vi "lj_start.vi"(6 "Period [ms]":i32=500 min=1 max=60000, 8 "error in (no error)":errorcluster, 10 "LabJackRes":T1, 11 "Handle In":i32) -> (0 "error out":errorcluster, 1 "NumReadAddresses":i32, 2 "ScansPerRead Out":i32, 3 "Handle Out":i32)   [LabVIEW 2025, in "LabJackEKG.lvlib"]
uses:
  LabJackEKG.lvlib
  Typedefs/LabJackGlobalResources.ctl
  Typedefs/CounterQueues.ctl
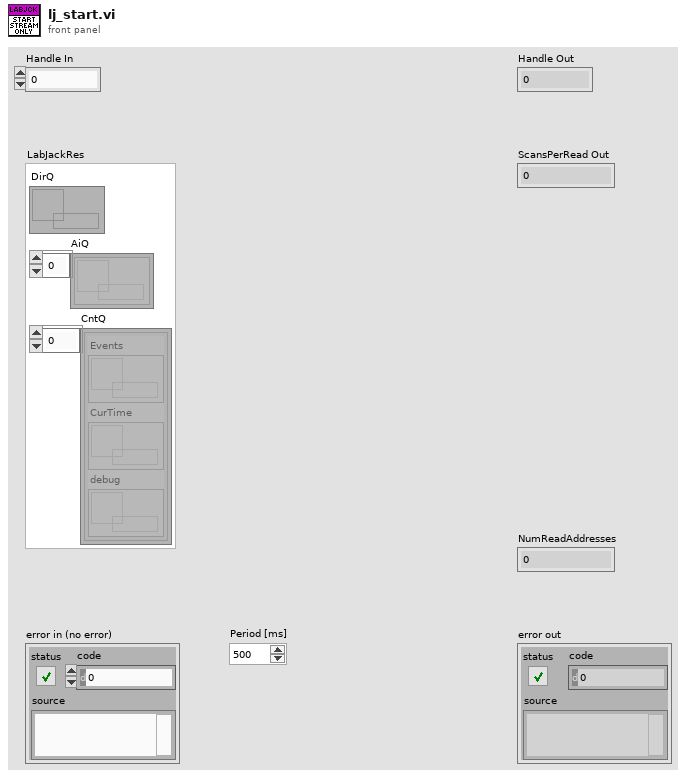
[diagram p1: front panel]
types:
  T1 = typedef "LabJackEKG.lvlib/LabJackGlobalResources.ctl" = cluster{"DirQ":refnum<queue>, "AiQ":refnum<queue>[], "CntQ":T2[]}
  T2 = typedef "LabJackEKG.lvlib/CounterQueues.ctl" = cluster{"Events":refnum<queue>, "CurTime":refnum<queue>, "debug":refnum<queue>}
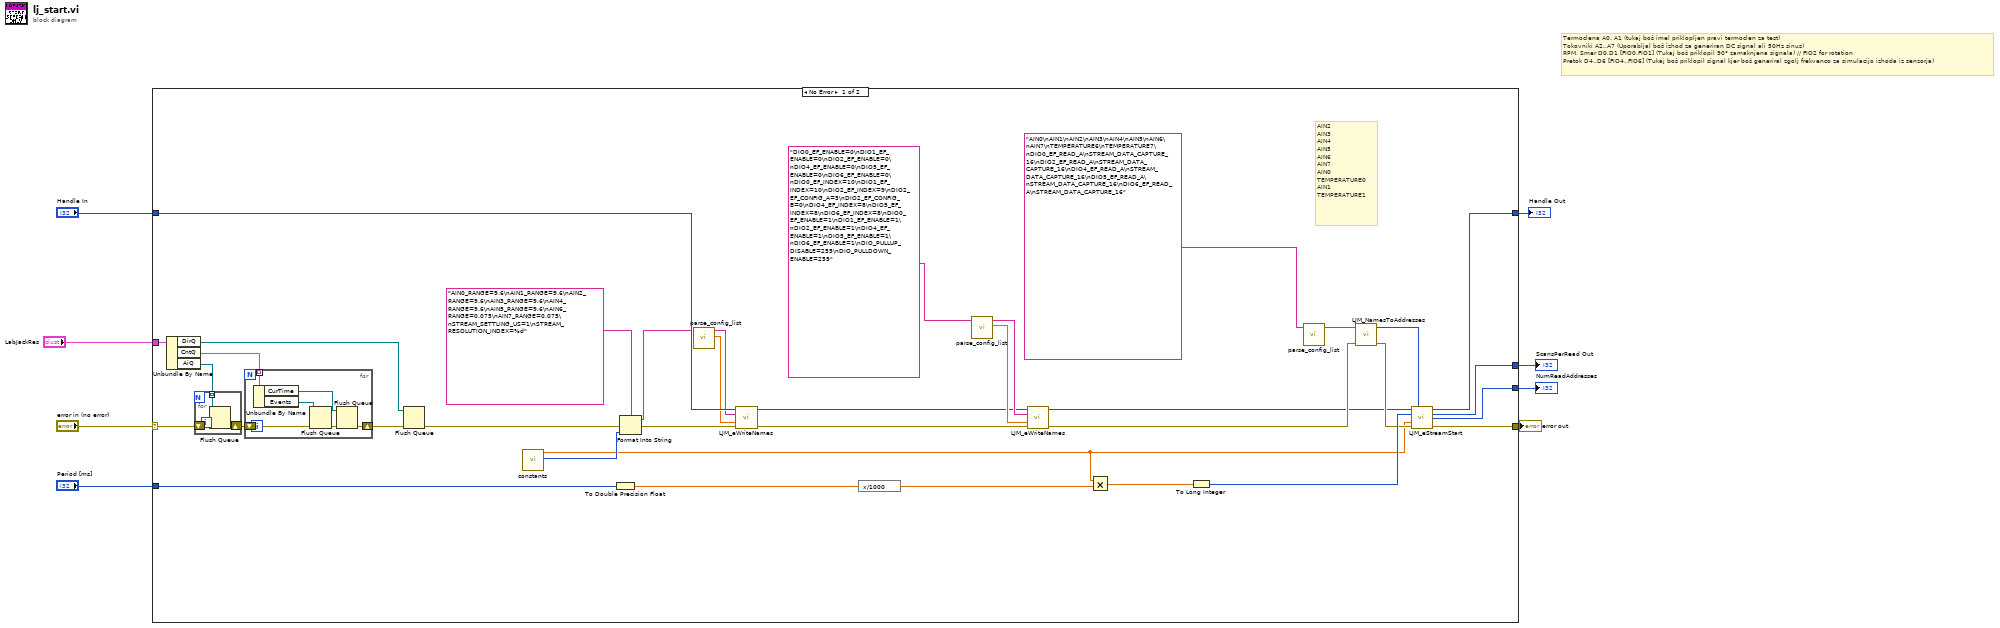
[diagram p0: block diagram]
diagram:
  # "Termoclena A0, A1 (tukaj boš imel priklopljen pravi termoclen za test)\nTokovniki A2..A7 (Uporabljal boš izhod za generiran DC signal ali 50Hz sinus)\nRPM, Smer D0,D1 [FIO0,FIO1] (Tukaj boš priklopil 90° zamaknjena signala) // FIO2 for rotation\nPretok D4..D6 [FIO4..FIO6] (Tukaj boš priklopil signal kjer boš generiral zgolj frekvenco za simulacijo izhoda iz senzorja)"
  n1 = case shown="No Error" "error in (no error)" {
    selector: "error in (no error)" -> [w44 w55]
    tunnel: [w41 w54] -> w8
    tunnel: "Handle In" -> [w43 w54]
    tunnel: [w42 w55] -> w5
    tunnel: [w39 _] -> w4
    tunnel: [w38 _] -> w3
    tunnel: "Period [ms]" -> [w37 _]
    tunnel: "LabJackRes" -> [w23 _]
    frame No Error {
      # "AIN2\nAIN3\nAIN4\nAIN5\nAIN6\nAIN7\nAIN0\nTEMPERATURE0\nAIN1\nTEMPERATURE1"
      n2 = Unbundle By Name(w23) -> ("DirQ"=w19:refnum<queue>, "CntQ"=w18:T2[], "AiQ"=w17:refnum<queue>[])
      n3 = for {
        shift-right: [w52] -> w22
        shift-left: w44 -> [w53]
        tunnel: w17 -> [w51] mode=indexing
        n4 = Flush Queue(queue=w51, error in (no error)=w53) -> (error out=w52:errorcluster)  [unwired: 2 out]
      }
      n5 = for {
        shift-right: [w46] -> w21
        shift-left: w22 -> [w50]
        tunnel: w18 -> [w48] mode=indexing
        n6 = Unbundle By Name(w48) -> ("CurTime"=w45:refnum<queue>, "Events"=w47:refnum<queue>)
        n7 = Flush Queue(queue=w47, error in (no error)=w50) -> (error out=w49:errorcluster)  [unwired: 2 out]
        n8 = Flush Queue(queue=w45, error in (no error)=w49) -> (error out=w46:errorcluster)  [unwired: 2 out]
      }
      n9 = Flush Queue(queue=w19, error in (no error)=w21) -> (error out=w20:errorcluster)  [unwired: 2 out]
      n10 = call "constants.vi"() -> ("Resolution Index"=w13:i32, "Sampling Frequency [Hz]"=w9:dbl)  [unwired: 10 in]
      n11 = To Double Precision Float(number=w37) -> (double precision float=w12:dbl)
      n12 = Format Into String(format string="AIN0_RANGE=9.6\nAIN1_RANGE=9.6\nAIN2_RANGE=9.6\nAIN3_RANGE=9.6\nAIN4_RANGE=9.6\nAIN5_RANGE=9.6\nAIN6_RANGE=0.075\nAIN7_RANGE=0.075\nSTREAM_SETTLING_US=1\nSTREAM_RESOLUTION_INDEX=%d" ("String"), error in=w20, w13) -> (resulting string=w14:string, error out=w16:errorcluster)  [unwired: 1 in]
      n13 = call "parse_config_list.vi"("String"=w14) -> ("Values"=w35:dbl[], "Names"=w36:string[])  [unwired: 9 in]
      n14 = call <vilib>:"LJM_eWriteNames.vi"("Handle In"=w43, "aNames"=w36, "aValuesIn"=w35, "error in"=w16) -> ("Handle Out"=w26:i32, "error out"=w27:errorcluster)  [unwired: 9 in, 1 out]
      n15 = expression code="x/1000"(w12) -> (w11:dbl)
      n16 = call "parse_config_list.vi"("String"="DIO0_EF_ENABLE=0\nDIO1_EF_ENABLE=0\nDIO2_EF_ENABLE=0\nDIO4_EF_ENABLE=0\nDIO5_EF_ENABLE=0\nDIO6_EF_ENABLE=0\nDIO0_EF_INDEX=10\nDIO1_EF_INDEX=10\nDIO2_EF_INDEX=9\nDIO2_EF_CONFIG_A=5\nDIO2_EF_CONFIG_B=0\nDIO4_EF_INDEX=8\nDIO5_EF_INDEX=8\nDIO6_EF_INDEX=8\nDIO0_EF_ENABLE=1\nDIO1_EF_ENABLE=1\nDIO2_EF_ENABLE=1\nDIO4_EF_ENABLE=1\nDIO5_EF_ENABLE=1\nDIO6_EF_ENABLE=1\nDIO_PULLUP_DISABLE=255\nDIO_PULLDOWN_ENABLE=255") -> ("Values"=w30:dbl[], "Names"=w29:string[])  [unwired: 9 in]
      n17 = call <vilib>:"LJM_eWriteNames.vi"("Handle In"=w26, "aNames"=w29, "aValuesIn"=w30, "error in"=w27) -> ("Handle Out"=w25:i32, "error out"=w28:errorcluster)  [unwired: 9 in, 1 out]
      n18 = Multiply(x=w9, y=w11) -> (x*y=w10:dbl)
      n19 = To Long Integer(number=w10) -> (32bit integer=w40:i32)
      n20 = call "parse_config_list.vi"("String"="AIN0\nAIN1\nAIN2\nAIN3\nAIN4\nAIN5\nAIN6\nAIN7\nTEMPERATURE6\nTEMPERATURE7\nDIO0_EF_READ_A\nSTREAM_DATA_CAPTURE_16\nDIO2_EF_READ_A\nSTREAM_DATA_CAPTURE_16\nDIO4_EF_READ_A\nSTREAM_DATA_CAPTURE_16\nDIO5_EF_READ_A\nSTREAM_DATA_CAPTURE_16\nDIO6_EF_READ_A\nSTREAM_DATA_CAPTURE_16") -> ("Names"=w33:string[])  [unwired: 9 in, 1 out]
      n21 = call <vilib>:"LJM_NamesToAddresses.vi"("error in"=w28, "aNames"=w33) -> ("error out"=w31:errorcluster, "aAddresses"=w32:i32[])  [unwired: 7 in, 1 out]
      n22 = call <vilib>:"LJM_eStreamStart.vi"("Handle In"=w25, "aScanList"=w32, "ScansPerRead"=w40, "ScanRate"=w9, "error in"=w31) -> ("Handle Out"=w41:i32, "ScansPerRead Out"=w38:i32, "NumReadAddresses"=w39:i32, "error out"=w42:errorcluster)  [unwired: 5 in, 2 out]
    }
    frame Error {
    }
  }
  "error out" <- w5
  "Handle Out" <- w8
  "ScansPerRead Out" <- w3
  "NumReadAddresses" <- w4
